vi "link_kf.vi"(6 "Reset":bool, 7 "Parameters":T3={"Stimulus"={"Type"=enum."Off", "Phase"=0.0, "Amplitude"=[], "Injection point"=enum."Total pose", "Closed loop"=FALSE, "Offset"=[], "Tip -> world"=FALSE, "Frequency"=0.0, "Length"=0.0}, "Goal Filter A"={"Speedup max"=0.0, "Speedup thresh"=0.0, "Speedup nonlin"=0.0, "Filters"=[]}, "Mode controls"={"Hold"=FALSE, "Cancellation"=FALSE, "Goal filter"=FALSE, "Trigger"=FALSE}, "Manipulator type"=enum."Current piezo", "Manipulator calibration"={"Tool offsets"=[[0.0, 0.0, 36200.0]], "Handle light calibration"=[], "Base pivots"=[], "Output pivots"=[], "Length center"=0.0, "Workspace height"=[], "Workspace diameter"=[0.0, 0.0, 36200.0], "Stack travel"=400.0, "Saturation pos"=375.0, "Inverse filters"=[], "Strut length"=0.0, "Tip light calibration"=[]}, "Network"={"Remote Host"="", "Send Status"=FALSE, "Send Port"=0, "Recv Commands"=FALSE, "Recv Port"=0}, "Goal Filter B"={"Speedup max"=0.0, "Speedup thresh"=0.0, "Speedup nonlin"=0.0, "Filters"=[]}, "Cancellation"={"KP"={"XY"=0.0, "Rxy"=0.0, "Z"=0.0, "Rz"=0.0}, "KI"=0.0, "KD"={"XY"=0.0, "Rxy"=0.0, "Z"=0.0, "Rz"=0.0}, "Max vel"=20.0, "Max acc"=0.001, "Int error limit"=3.0, "RCM gain"=0.0, "Bypass"=FALSE, "Degraded gain"=0.0}, "Transition time"=0.0, "Estimation"={"Link"={"Measure noise"=[], "Process noise"=[], "Alt process noise"=[], "Alt turnoff cycles"=20, "Innovation limit"=[], "Residue threshold"=0.0, "Enable"=FALSE}, "Handle"={"Measure noise"=[], "Process noise"=[], "State limits"=[], "Innovation limit"=[], "Prediction Lookahead"=0.0, "Enable"=FALSE}}} {"Transition time" format="%_3f"; "Cancellation"."Degraded gain" min=0 max=1 step=0.1 format="%#_3p"; "Cancellation"."RCM gain" min=0 max=1 step=0.1 format="%#_3p"; "Cancellation"."KD"."Rz" min=-1 max=1 step=0.01 format="%#_3p"; "Cancellation"."KD"."Rxy" min=-1 max=1 step=0.01 format="%#_3p"; "Cancellation"."KD"."Z" min=-1 max=1 step=0.01 format="%#_3p"; "Cancellation"."KD"."XY" min=-1 max=1 step=0.01 format="%#_3p"; "Cancellation"."KI" min=0 max=1 step=0.01 format="%#_3p"; "Cancellation"."KP"."Rz" min=-1 max=1 step=0.01 format="%#_3p"; "Cancellation"."KP"."Rxy" min=-1 max=1 step=0.01 format="%#_3p"; "Cancellation"."KP"."Z" min=-1 max=1 step=0.01 format="%#_3p"; "Cancellation"."KP"."XY" min=-1 max=1 step=0.01 format="%#_3p"; "Cancellation"."Max acc" format="%#_3p"; "Goal Filter B"."Filters"."V limit range" format="%_3p"; "Goal Filter B"."Filters"."V limit" format="%_3p"; "Goal Filter B"."Filters"."Upper Q" format="%_3f"; "Goal Filter B"."Filters"."Upper Fc" format="%_3p"; "Goal Filter B"."Filters"."Lower Q" format="%_3f"; "Goal Filter B"."Filters"."Scale factor" format="%_3f"; "Goal Filter B"."Filters"."Lower Fc" format="%_3p"; "Goal Filter B"."Speedup nonlin" format="%_3p"; "Goal Filter B"."Speedup thresh" format="%_3p"; "Goal Filter B"."Speedup max" format="%_3p"; "Manipulator calibration"."Tip light calibration" format="%#.1f"; "Manipulator calibration"."Strut length" format="%#_4p"; "Manipulator calibration"."Saturation pos" format="%#.1f"; "Manipulator calibration"."Stack travel" format="%#.1f"; "Manipulator calibration"."Length center" format="%#_4p"; "Manipulator calibration"."Output pivots" format="%#_6f"; "Manipulator calibration"."Base pivots" format="%#_6f"; "Manipulator calibration"."Handle light calibration" format="%#.1f"; "Goal Filter A"."Filters"."V limit range" format="%_3p"; "Goal Filter A"."Filters"."V limit" format="%_3p"; "Goal Filter A"."Filters"."Upper Q" format="%_3f"; "Goal Filter A"."Filters"."Upper Fc" format="%_3p"; "Goal Filter A"."Filters"."Lower Q" format="%_3f"; "Goal Filter A"."Filters"."Scale factor" format="%_3f"; "Goal Filter A"."Filters"."Lower Fc" format="%_3p"; "Goal Filter A"."Speedup nonlin" format="%_3p"; "Goal Filter A"."Speedup thresh" format="%_3p"; "Goal Filter A"."Speedup max" format="%_3p"; "Stimulus"."Length" min=0.0 max=100.0 step=100.0 format="%#_4p"; "Stimulus"."Frequency" min=0.0 step=100.0 format="%#_4g"; "Stimulus"."Offset" format="%#_3p"; "Stimulus"."Amplitude" format="%#_3p"; "Stimulus"."Phase" min=-180.0 max=360.0 step=100.0 format="%#.2f"}, 9 "Last output command":sgl[](array[numeric]), 11 "Raw link position":sgl[](array[numeric])) -> (0 "Position residue":sgl[](array[numeric]) format="%#_3p", 1 "Link rates":sgl[](array[numeric]) format="%#_3p", 3 "KF link position":sgl[](array[numeric]) format="%#_3g", 5 "Degraded":bool[](array[boolean]))   [LabVIEW 2014]
uses:
  utilities/labview/kalman_filter.ctl
  <vilib>/Analysis/Matrix/Datatypes/RealMatrix.ctl
  testing/Micron params.ctl
  testing/stimulus.ctl
  testing/injection_point.ctl
  filtering/goal_loop_parms.ctl
  testing/mode_conrols.ctl
  testing/manipulator_cal.ctl
  asap/labview/testing/probe_calibration.ctl
  host/network_params.ctl
  sq_control_params.ctl
  decoupled_gain.ctl
  estimation_controls.ctl
  <vilib>/Analysis/Matrix/Numeric/Conversions/Array To Matrix - RA.vi
  <vilib>/Analysis/Matrix/NI_Matrix.lvlib
panel:
  in  "Alt filter turnoff counter":i32[](array[numeric])
  in  "Late turnoff":bool=TRUE
  out "Alt position residue":sgl[](array[numeric]) format="%#_3p"
  in  "Alt u filter":T1={"A"=[], "B"=[], "H"=[], "Q"=[], "R"=[], "x"=[], "P"=[], "x lim"=[], "y lim"=[], "K"=[], "Converge count"=-1} {"K" format="%#_3g"; "y lim" format="%#_3g"; "x lim" format="%#_3g"; "P" format="%#_3g"; "H" format="%#_3g"; "x" format="%#_3g"; "Q" format="%#_3g"; "R" format="%#_3g"; "B" format="%#_3g"; "A" format="%#_3g"}
  out "Rate filter position":sgl[](array[numeric]) format="%#_3g"
  out "Rate residue":sgl[](array[numeric]) format="%#_3p"
  in  "Rate filter":T1={"A"=[], "B"=[], "H"=[], "Q"=[], "R"=[], "x"=[], "P"=[], "x lim"=[], "y lim"=[], "K"=[], "Converge count"=-1} {"K" format="%#_3g"; "y lim" format="%#_3g"; "x lim" format="%#_3g"; "P" format="%#_3g"; "H" format="%#_3g"; "x" format="%#_3g"; "Q" format="%#_3g"; "R" format="%#_3g"; "B" format="%#_3g"; "A" format="%#_3g"}
  in  "u filter":T1={"A"=[], "B"=[], "H"=[], "Q"=[], "R"=[], "x"=[], "P"=[], "x lim"=[], "y lim"=[], "K"=[], "Converge count"=-1} {"K" format="%#_3g"; "y lim" format="%#_3g"; "x lim" format="%#_3g"; "P" format="%#_3g"; "H" format="%#_3g"; "x" format="%#_3g"; "Q" format="%#_3g"; "R" format="%#_3g"; "B" format="%#_3g"; "A" format="%#_3g"}
  # "Control authority is degraded on this axis (high residue.)  Higher process noise reduces phase lead."
  # "Debugging"
  # "Feedforward filter with higher process noise for when an axis is misbehaving."
  # "Six 2-state filters (position, velocity), one for each axis."
  # "Six one-state filters (position), with command feedforward."
  # "Local variables:"
  # "It seems it isn't coherent to have both an estimated rate and a rate control input in the same filter, so instead we have two filters, one with a command input and no rate state, and another with no input and with rate estimation."
  # "Constant velocity\ntransition matrix."
  # "Constant position"
  # "state covariance"
  # "Command\naffects \nposition"
  # "No command input"
  # "Process noise for position and velocity."
  # "The measurement is position"
  # "Link position measurement noise."
  # "Number of cycles since the last time we exceeded the residue theshold, per axis."
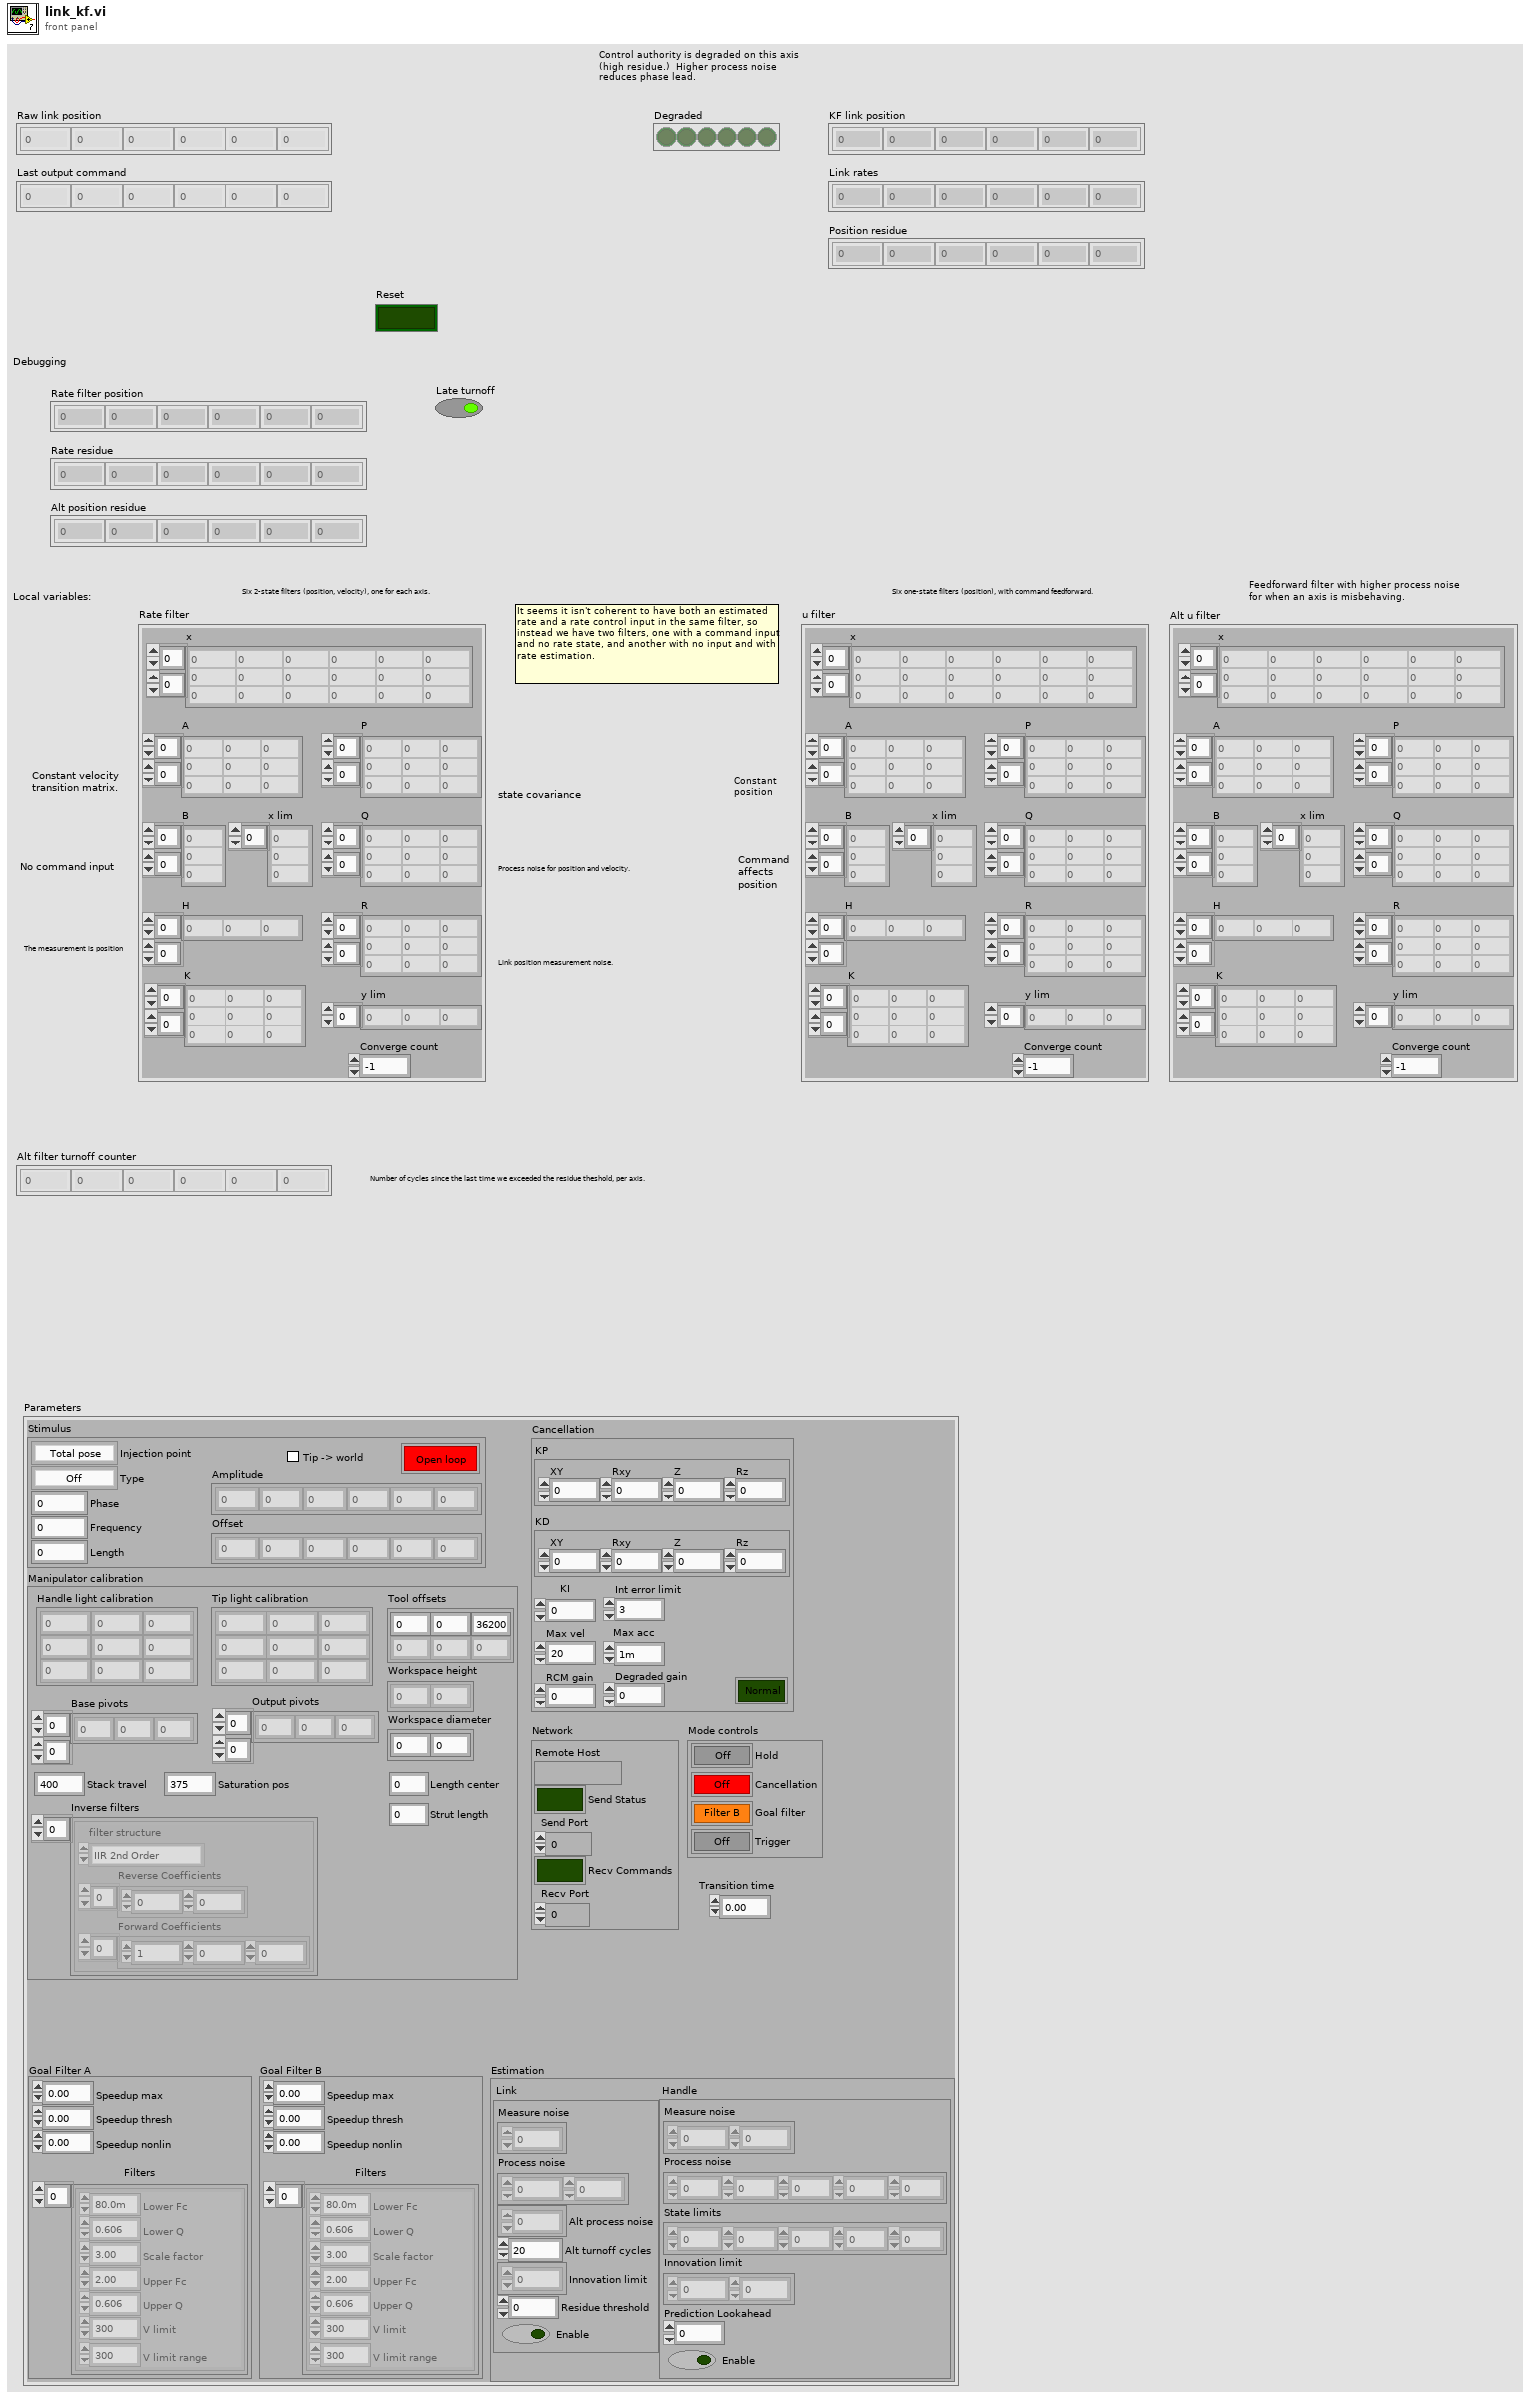
[diagram p1: front panel]
types:
  T1 = typedef "kalman_filter.ctl" = cluster{"A":T2, "B":T2, "H":T2, "Q":T2, "R":T2, "x":T2, "P":T2, "x lim":dbl[], "y lim":dbl[], "K":T2, "Converge count":i32}
  T2 = typedef "NI_Matrix.lvlib/RealMatrix.ctl" = dbl[][]
  T3 = typedef "Micron params.ctl" = cluster{"Stimulus":T4, "Goal Filter A":T6, "Mode controls":T7, "Manipulator type":enum16{"Current piezo", "Voltage piezo"}, "Manipulator calibration":T8, "Network":T10, "Goal Filter B":T6, "Cancellation":T11, "Transition time":sgl, "Estimation":T13}
  T4 = typedef "stimulus.ctl" = cluster{"Type":enum16{"Off", "Step", "Sine", "Triangle", "Arbitrary"}, "Phase":dbl, "Amplitude":sgl[], "Injection point":T5, "Closed loop":bool, "Offset":sgl[], "Tip -> world":bool, "Frequency":dbl, "Length":dbl}
  T5 = typedef "injection_point.ctl" = enum16{"Total pose", "V limiter", "Goal ", "Link position", "KF link position", "Inverse kin", "Link goal", "Link error", "Controller", "Output", "Drive", "Light"}
  T6 = typedef "goal_loop_parms.ctl" = cluster{"Speedup max":sgl, "Speedup thresh":sgl, "Speedup nonlin":sgl, "Filters":cluster{"Lower Fc":sgl, "Lower Q":sgl, "Scale factor":sgl, "Upper Fc":sgl, "Upper Q":sgl, "V limit":sgl, "V limit range":sgl}[]}
  T7 = typedef "mode_conrols.ctl" = cluster{"Hold":bool, "Cancellation":bool, "Goal filter":bool, "Trigger":bool}
  T8 = typedef "manipulator_cal.ctl" = cluster{"Tool offsets":sgl[][], "Handle light calibration":T9, "Base pivots":sgl[][], "Output pivots":sgl[][], "Length center":sgl, "Workspace height":sgl[], "Workspace diameter":sgl[], "Stack travel":sgl, "Saturation pos":sgl, "Inverse filters":cluster{"filter structure":enum32{"IIR 2nd Order", "IIR 4th Order"}, "Reverse Coefficients":dbl[], "Forward Coefficients":dbl[]}[], "Strut length":sgl, "Tip light calibration":T9}
  T9 = typedef "probe_calibration.ctl" = sgl[][]
  T10 = typedef "network_params.ctl" = cluster{"Remote Host":string, "Send Status":bool, "Send Port":u16, "Recv Commands":bool, "Recv Port":u16}
  T11 = typedef "sq_control_params.ctl" = cluster{"KP":T12, "KI":sgl, "KD":T12, "Max vel":sgl, "Max acc":sgl, "Int error limit":sgl, "RCM gain":sgl, "Bypass":bool, "Degraded gain":sgl}
  T12 = typedef "decoupled_gain.ctl" = cluster{"XY":sgl, "Rxy":sgl, "Z":sgl, "Rz":sgl}
  T13 = typedef "estimation_controls.ctl" = cluster{"Link":cluster{"Measure noise":dbl[], "Process noise":dbl[], "Alt process noise":dbl[], "Alt turnoff cycles":i32, "Innovation limit":dbl[], "Residue threshold":dbl, "Enable":bool}, "Handle":cluster{"Measure noise":dbl[], "Process noise":dbl[], "State limits":dbl[], "Innovation limit":dbl[], "Prediction Lookahead":sgl, "Enable":bool}}
  T14 = cluster{"Measure noise":dbl[], "Process noise":dbl[], "Alt process noise":dbl[], "Alt turnoff cycles":i32, "Innovation limit":dbl[], "Residue threshold":dbl, "Enable":bool}
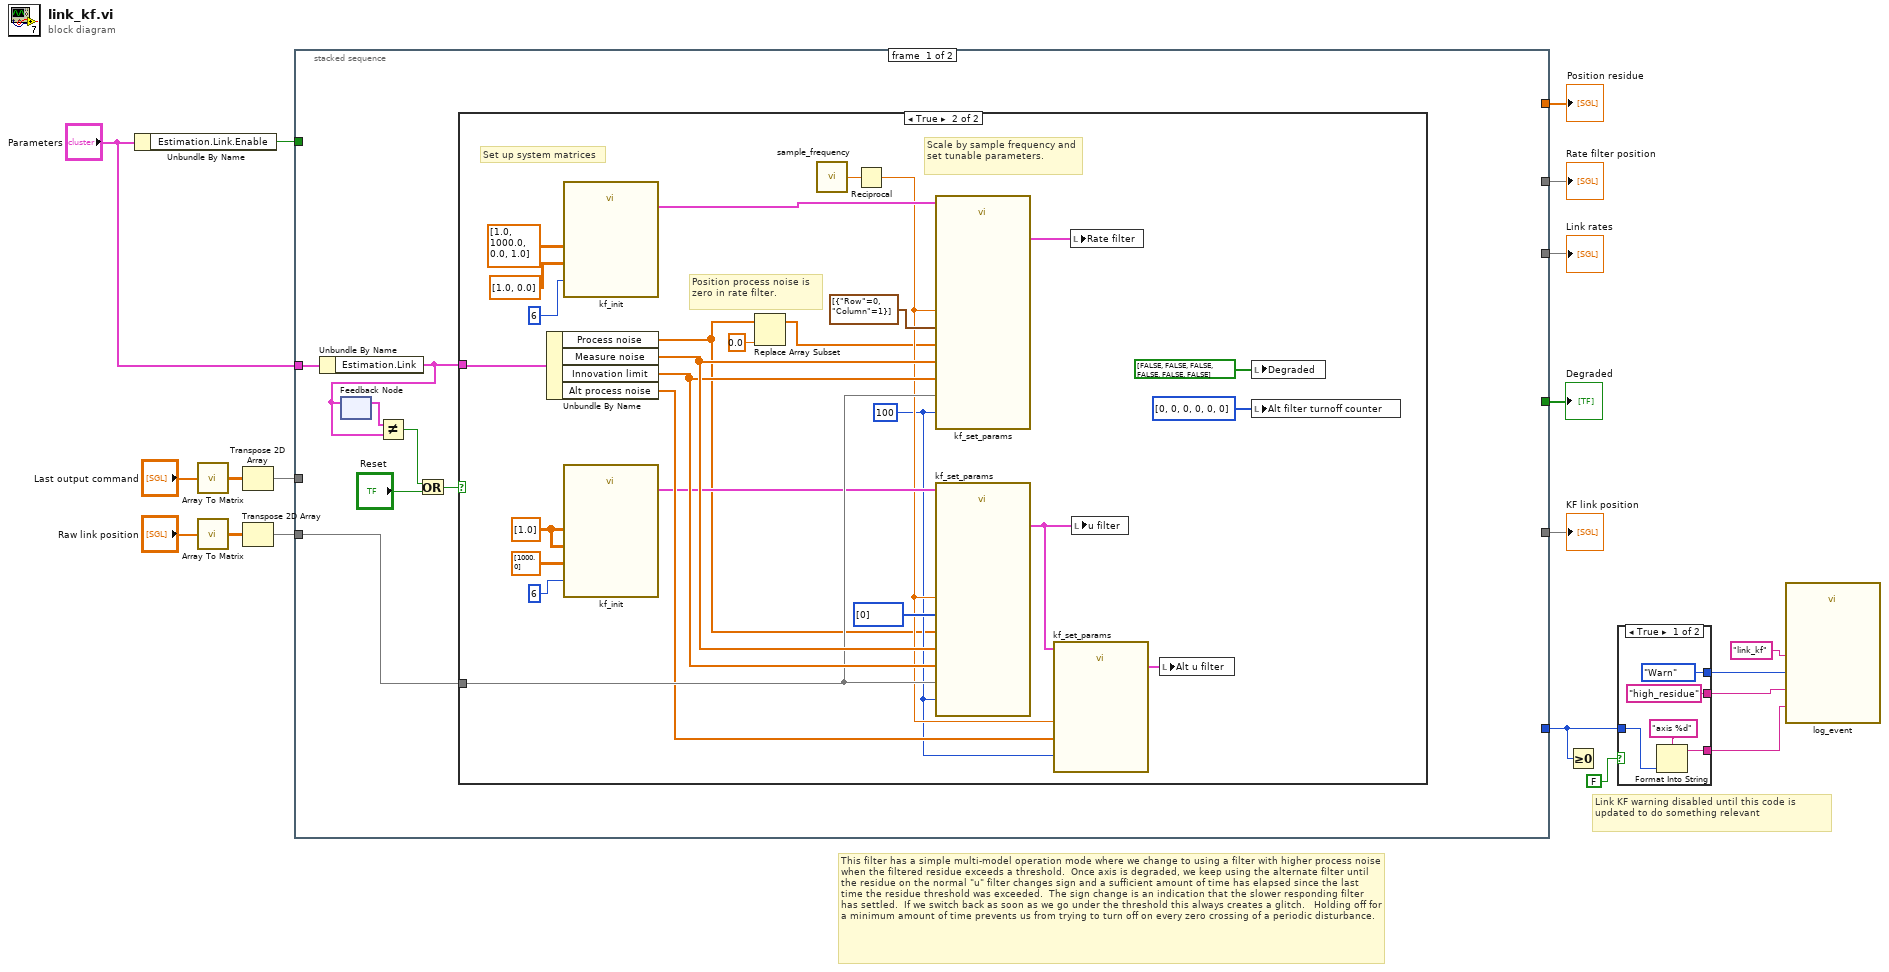
[diagram p0: block diagram]
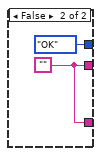
[diagram p2: hidden frame]
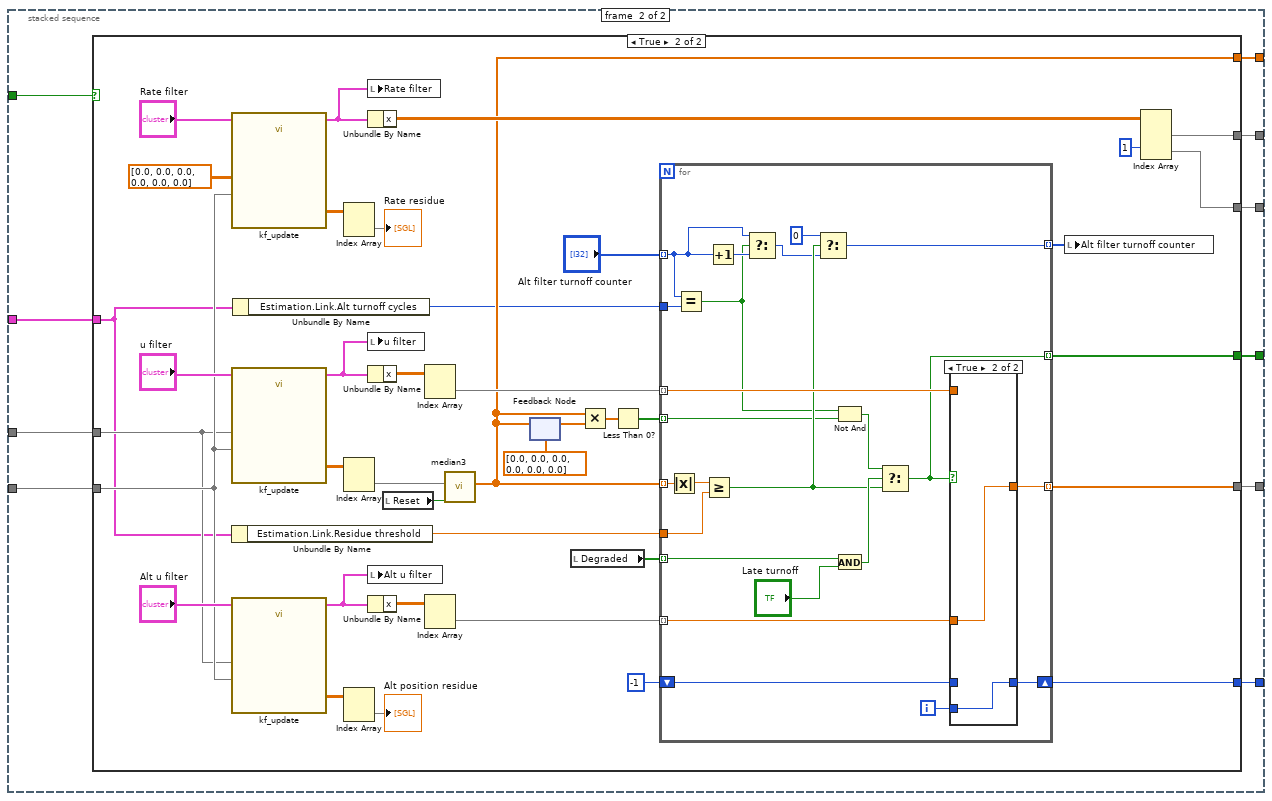
[diagram p4: hidden frame]
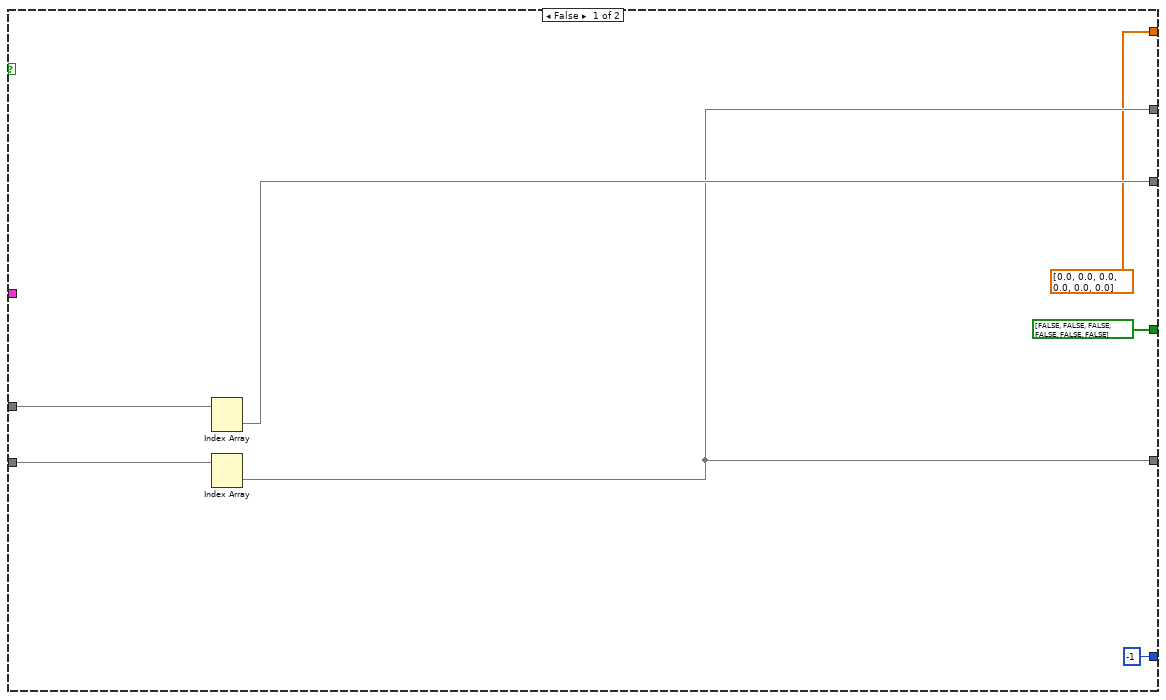
[diagram p5: hidden frame]
diagram:
  # "Link KF warning disabled until this code is updated to do something relevant"
  # "This filter has a simple multi-model operation mode where we change to using a filter with higher process noise when the filtered residue exceeds a threshold.  Once axis is degraded, we keep using the alternate filter until the residue on the normal \"u\" filter changes sign and a sufficient amount of time has elapsed since the last time the residue threshold was exceeded.  The sign change is an indication that the slower responding filter has settled.  If we switch back as soon as we go under the threshold this always creates a glitch.   Holding off for a minimum amount of time prevents us from trying to turn off on every zero crossing of a periodic disturbance."
  n1 = Unbundle By Name("Parameters") -> ("Estimation.Link.Enable"=w15:bool)
  n2 = call-poly <vilib>:"Array To Matrix.vi"("Real 1D Array"="Last output command") -> ("Real Matrix (Column Vector)"=w14:T2)
  n3 = call-poly <vilib>:"Array To Matrix.vi"("Real 1D Array"="Raw link position") -> ("Real Matrix (Column Vector)"=w13:T2)
  n4 = Transpose 2D Array(2D array=w14) -> (transposed array=w12:T2)
  n5 = Transpose 2D Array(2D array=w13) -> (transposed array=w11:T2)
  n6 = stacked-sequence {
    tunnel: w11 -> [w26 w62]
    tunnel: [_ w61] -> w19
    tunnel: [_ w60] -> w17
    tunnel: w12 -> [_ w59]
    tunnel: [_ w58] -> w18
    tunnel: "Parameters" -> [w23 w56]
    tunnel: w15 -> [_ w57]
    tunnel: [_ w55] -> w8
    tunnel: [_ w54] -> w7
    tunnel: [_ w53] -> w2
    frame #0 {
      n7 = Unbundle By Name(w23) -> ("Estimation.Link"=w20:T14)
      n8 = feedback #1() -> (w24:T14)  [unwired: 1 in]
      n9 = feedback-in #1(w20) -> ()
      n10 = Not Equal?(x=w24, y=w20) -> (x != y?=w25:bool)
      n11 = Or(x=w25, y="Reset") -> (x .or. y?=w22:bool)
      n12 = case shown="True" w22 {
        tunnel: w20 -> [_ w51]
        tunnel: w26 -> [_ w45]
        frame False {
        }
        frame True {
          w30 = 100 ("Converge count")
          w37 = T2 [[1.0]] ("A")
          # "Position process noise is zero in rate filter."
          # "Set up system matrices"
          # "Scale by sample frequency and set tunable parameters."
          n13 = Unbundle By Name(w51) -> ("Process noise"=w29:dbl[], "Measure noise"=w48:dbl[], "Innovation limit"=w47:dbl[], "Alt process noise"=w43:dbl[])
          n14 = call "kf_init.vi"("A"=T2 [[1.0, 1000.0], [0.0, 1.0]], "H"=T2 [[1.0, 0.0]] ("B"), "x columns"=6) -> ("KF out"=w39:T1)  [unwired: 12 in]
          n15 = call "kf_init.vi"("A"=w37, "B"=T2 [[1000.0]] ("A"), "H"=w37, "x columns"=6) -> ("KF out"=w35:T1)  [unwired: 11 in]
          n16 = Replace Array Subset(array=w29, new element=0.0 ("new element/subarray")) -> (w27:dbl[])  [unwired: 1 in]
          n17 = call "sample_frequency.vi"() -> ("Sample frequency"=w52:dbl)
          n18 = Reciprocal(x=w52) -> (1/x=w33:dbl)
          n19 = call "kf_set_params.vi"("KF in"=w39, "Innovation limits"=w47, "Process noise"=w27, "Initial input"=w45, "Measurement noise"=w48, "A scale indices"=cluster{"Row":i32, "Column":i32}[] [{"Row"=0, "Column"=1}], "Scale factor"=w33, "Converge count"=w30) -> ("KF out"=w46:T1)  [unwired: 11 in]
          n20 = call "kf_set_params.vi"("KF in"=w35, "Innovation limits"=w47, "Process noise"=w29, "Initial input"=w45, "Measurement noise"=w48, "B scale indices"=i32[] [0], "Scale factor"=w33, "Converge count"=w30) -> ("KF out"=w44:T1)  [unwired: 11 in]
          n21 = call "kf_set_params.vi"("KF in"=w44, "Process noise"=w43, "Scale factor"=w33, "Converge count"=w30) -> ("KF out"=w34:T1)  [unwired: 15 in]
          n22 = local write "Rate filter"(w46) -> ()
          n23 = local write "u filter"(w44) -> ()
          n24 = local write "Alt u filter"(w34) -> ()
          n25 = local write "Degraded"(bool[] [FALSE, FALSE, FALSE, FALSE, FALSE, FALSE]) -> ()
          n26 = local write "Alt filter turnoff counter"(i32[] [0, 0, 0, 0, 0, 0] ("Out")) -> ()
        }
      }
    }
    frame #1 {
      n27 = case shown="True" w57 {
        tunnel: w62 -> [w67 w91]
        tunnel: [w66 w83] -> w61
        tunnel: [w66 w105] -> w60
        tunnel: w59 -> [w69 w90]
        tunnel: [w68 w98] -> w58
        tunnel: w56 -> [_ w71]
        tunnel: [bool[] [FALSE, FALSE, FALSE, FALSE, FALSE, FALSE] w81] -> w55
        tunnel: [sgl[] [0.0, 0.0, 0.0, 0.0, 0.0, 0.0] ("Out") w73] -> w54
        tunnel: [-1 w74] -> w53
        frame False {
          n28 = Index Array(array=w69) -> (element=w68:dbl[])  [unwired: 2 in]
          n29 = Index Array(array=w67) -> (element=w66:dbl[])  [unwired: 2 in]
        }
        frame True {
          n30 = call "kf_update.vi"("z"=w91, "u"=T2 [[0.0, 0.0, 0.0, 0.0, 0.0, 0.0]], "KF in"="Rate filter") -> ("y"=w100:T2, "KF out"=w102:T1)  [unwired: 7 in]
          n31 = call "kf_update.vi"("z"=w91, "u"=w90, "KF in"="u filter") -> ("y"=w108:T2, "KF out"=w107:T1)  [unwired: 7 in]
          n32 = Unbundle By Name(w71) -> ("Estimation.Link.Residue threshold"=w88:dbl)
          n33 = call "kf_update.vi"("z"=w91, "u"=w90, "KF in"="Alt u filter") -> ("y"=w93:T2, "KF out"=w89:T1)  [unwired: 7 in]
          n34 = Unbundle By Name(w71) -> ("Estimation.Link.Alt turnoff cycles"=w70:i32)
          n35 = Index Array(array=w100) -> (element=→"Rate residue":dbl[])  [unwired: 2 in]
          n36 = Index Array(array=w108) -> (element=w85:dbl[])  [unwired: 2 in]
          n37 = Index Array(array=w93) -> (element=→"Alt position residue":dbl[])  [unwired: 2 in]
          n38 = local write "Rate filter"(w102) -> ()
          n39 = Unbundle By Name(w102) -> ("x"=w103:T2)
          n40 = local write "u filter"(w107) -> ()
          n41 = Unbundle By Name(w107) -> ("x"=w106:T2)
          n42 = local write "Alt u filter"(w89) -> ()
          n43 = Unbundle By Name(w89) -> ("x"=w95:T2)
          n44 = local read "Reset"() -> (w84:bool)
          n45 = Index Array(array=w106) -> (element=w87:dbl[])  [unwired: 2 in]
          n46 = Index Array(array=w95) -> (element=w86:dbl[])  [unwired: 2 in]
          n47 = call "median3.vi"("Reset"=w84, "In"=w85) -> ("Out"=w73:sgl[])  [unwired: 9 in]
          n48 = feedback-in #2(w73) -> ()
          n49 = feedback #2(sgl[] [0.0, 0.0, 0.0, 0.0, 0.0, 0.0] ("Out")) -> (w78:sgl[])
          n50 = local read "Degraded"() -> (w79:bool[])
          n51 = Multiply(x=w73, y=w78) -> (x*y=w76:sgl[])
          n52 = Less Than 0?(x=w76) -> (x < 0?=w80:bool[])
          n53 = for {
            tunnel: w73 -> [w131] mode=indexing
            tunnel: w88 -> [w129]
            tunnel: w87 -> [w123] mode=indexing
            tunnel: w86 -> [w127] mode=indexing
            tunnel: [w128] -> w83 mode=indexing
            shift-right: [w126] -> w74
            shift-left: -1 -> [w124]
            tunnel: [w122] -> w81 mode=indexing
            tunnel: w80 -> [w110] mode=indexing
            tunnel: w79 -> [w120] mode=indexing
            tunnel: "Alt filter turnoff counter" -> [w114] mode=indexing
            tunnel: [w116] -> w75 mode=indexing
            tunnel: w70 -> [w115]
            i -> [w125]
            n54 = Absolute Value(x=w131) -> (abs(x)=w130:sgl)
            n55 = Equal?(x=w114, y=w115) -> (x = y?=w109:bool)
            n56 = Greater Or Equal?(x=w130, y=w129) -> (x >= y?=w118:bool)
            n57 = Increment(x=w114) -> (x+1=w113:i32)
            n58 = Select(t=w114, s=w109, f=w113) -> (s? t:f=w112:i32)
            n59 = Select(t=0, s=w118, f=w112) -> (s? t:f=w116:i32)
            n60 = Not And(1:w110, 2:w109) -> (0:w111:bool)
            n61 = And(x=w120, y="Late turnoff") -> (x .and. y?=w119:bool)
            n62 = Select(t=w111, s=w119, f=w118) -> (s? t:f=w122:bool)
            n63 = case shown="True" w122 {
              tunnel: [w132 w135] -> w128
              tunnel: w127 -> [_ w135]
              tunnel: [w133 w134] -> w126
              tunnel: w125 -> [_ w134]
              tunnel: w124 -> [w133 _]
              tunnel: w123 -> [w132 _]
              frame False {
              }
              frame True {
              }
            }
          }
          n64 = local write "Alt filter turnoff counter"(w75) -> ()
          n65 = Index Array(array=w103, index (row) #2=1 ("index (row)")) -> (element #1=w105:dbl[], element #2=w98:dbl[])  [unwired: 3 in]
        }
      }
    }
  }
  "KF link position" <- w19
  "Link rates" <- w18
  "Rate filter position" <- w17
  "Degraded" <- w8
  "Position residue" <- w7
  n66 = Greater Or Equal To 0?(x=w2) -> ()  [unwired: 1 out]
  n67 = case shown="True" FALSE {
    tunnel: [enum16{"OK", "Debug", "Warn", "Error"}."Warn" ("Severity") enum16{"OK", "Debug", "Warn", "Error"}."OK" ("Severity")] -> w3
    tunnel: ["high_residue" ("State") w141] -> w4
    tunnel: w2 -> [w137 _]
    tunnel: [w136 w141] -> w5
    frame True {
      n68 = Format Into String(format string="axis %d", w137) -> (resulting string=w136:string)  [unwired: 2 in, 1 out]
    }
    frame False {
      w141 = "" ("State")
    }
  }
  n69 = call "log_event.vi"("Message"=w5, "State"=w4, "Facility"="link_kf", "Severity"=w3) -> ()  [unwired: 7 in, 1 out]
